vi "sound.vi"() -> ()   [LabVIEW 2010]
uses:
  <vilib>/sound2/lvsound2.llb/Sound Data Format.ctl
  <vilib>/sound2/lvsound2.llb/Sound Output Task ID.ctl
panel:
  in  "milliseconds to wait":u32
  in  "Tab Control":enum32{"Sound"}(tab)
  in  "Sound Controls":T2={"device ID"=0, "sound format"={"sample rate (S/s)"=44000.0, "number of channels"=2, "bits per sample"=16}, "time (ms)"=200.0}
  in  "Sound?":bool
  in  "Frecuencia":dbl
  out "Waveform Sound":waveform(dbl)(graph)
  out "tiempo transcurrido(ms)":u32
  in  "stop":bool
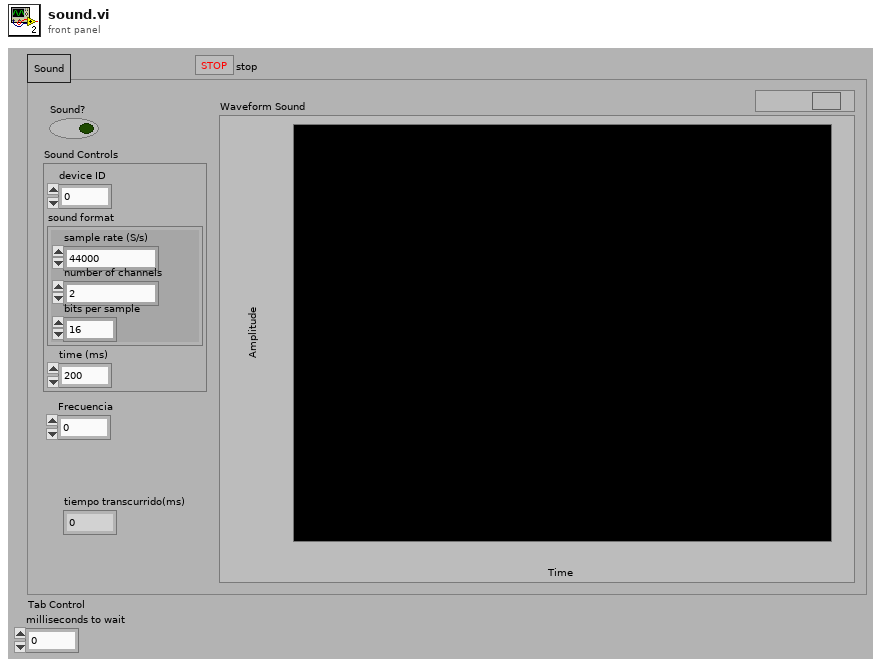
[diagram p1: front panel]
types:
  T1 = typedef "Sound Data Format.ctl" = cluster{"sample rate (S/s)":dbl, "number of channels":i32, "bits per sample":i32}
  T2 = cluster{"device ID":u32, "sound format":T1, "time (ms)":dbl}
  T3 = typedef "Sound Output Task ID.ctl" = u32
  T4 = cluster{"task ID":T3, "error":errorcluster, "sound format":T1}
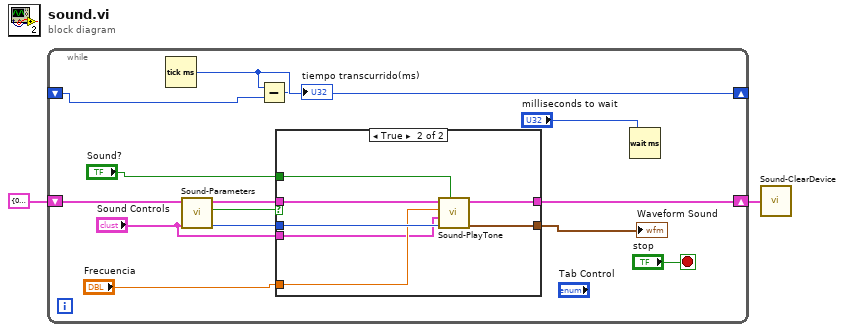
[diagram p0: block diagram]
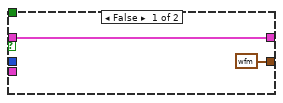
[diagram p2: hidden frame]
diagram:
  n1 = while {
    shift-right: [w12] -> w1
    shift-left: T4 {"task ID"=0, "error"={"status"=TRUE, "code"=0, "source"=""}, "sound format"={"sample rate (S/s)"=0.0, "number of channels"=0, "bits per sample"=0}} ("Sound Device OUT") -> [w11]
    shift-right: [w5] -> _
    shift-left: _ -> [w6]
    stop <- "stop" stop-if-true
    n2 = Tick Count (ms)() -> (millisecond timer value=w5:u32)
    n3 = call "Sound-Parameters.vi"("Sound Controls"="Sound Controls", "Sound Device IN"=w11) -> ("#samples"=w13:u32, "En funcionamiento?"=w10:bool, "Sound Device OUT"=w14:T4)  [unwired: 3 in]
    n4 = Subtract(x=w5, y=w6) -> (x-y=→"tiempo transcurrido(ms)":u32)
    n5 = case shown="True" w10 {
      tunnel: [waveform(dbl) {"t0"=timestamp(0 s since 1904-01-01), "dt"=1.0, "Y"=[]} ("Waveform") w25] -> w15
      tunnel: w14 -> [w18 w24]
      tunnel: w13 -> [_ w23]
      tunnel: [w18 w22] -> w12
      tunnel: "Sound?" -> [_ w21]
      tunnel: "Frecuencia" -> [_ w20]
      tunnel: "Sound Controls" -> [_ w19]
      frame False {
      }
      frame True {
        n6 = call "Sound-PlayTone.vi"("sound?"=w21, "# samples"=w23, "Sound Controls"=w19, "Frecuencia"=w20, "Sound Device IN"=w24) -> ("Waveform"=w25:waveform(dbl), "Sound Device OUT"=w22:T4)  [unwired: 3 in]
      }
    }
    "Waveform Sound" <- w15
    n7 = Wait (ms)(milliseconds to wait="milliseconds to wait") -> ()  [unwired: 1 out]
  }
  n8 = call "Sound-ClearDevice.vi"("Sound Device OUT"=w1) -> ()
